vi "ChassisSetSpeeds.vi"(9 "DriveSpeedRight":dbl, 10 "DriveSpeedLeft":dbl) -> ()   [LabVIEW 2014, in "ChassisLib.lvlib"]
uses:
  ChassisLib.lvlib
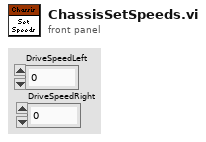
[diagram p1: front panel]
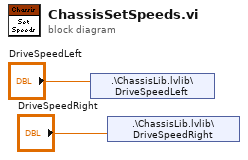
[diagram p0: block diagram]
diagram:
  n1 = shared-variable ".\\ChassisLib.lvlib\\DriveSpeedLeft"("DriveSpeedLeft") -> ()  [unwired: 1 in, 1 out]
  n2 = shared-variable ".\\ChassisLib.lvlib\\DriveSpeedRight"("DriveSpeedRight") -> ()  [unwired: 1 in, 1 out]
